vi "FeedbackDecode_UnpackPupilInfo.vi"(8 "ErrorIn":errorcluster, 11 "MSGPackStr":string="ˆ¥topic¥pupilªconfidenceË\u0000\u0000\u0000\u0000\u0000\u0000\u0000\u0000§ellipseƒ¦center’Ë\u0000\u0000\u0000\u0000\u0000\u0000\u0000\u0000Ë\u0000\u0000\u0000\u0000\u0000\u0000\u0000\u0000¤axes’Ë\u0000\u0000\u0000\u0000\u0000\u0000\u0000\u0000Ë\u0000\u0000\u0000\u0000\u0000\u0000\u0000\u0000¥angleËÀV€\u0000\u0000\u0000\u0000\u0000¨diameterË\u0000\u0000\u0000\u0000\u0000\u0000\u0000\u0000¨norm_pos’Ë\u0000\u0000\u0000\u0000\u0000\u0000\u0000\u0000Ë?ð\u0000\u0000\u0000\u0000\u0000\u0000©timestampË@µïXf¡\u001eÉ¦method¦2d c++¢id\u0000") -> (0 "ErrorOut":errorcluster, 3 "PupilClust":T1, 4 "Pupil2d":bool)   [LabVIEW 2020]
uses:
  MsgPack_LabVIEW-master/MsgPack.lvlib
panel:
  out "EmptyCnt":i32
  out "Array":variant[](array[variant])
  # "conf 8,\ndia3d 12,\nts 10\ndia 18\nmdlconf 24"
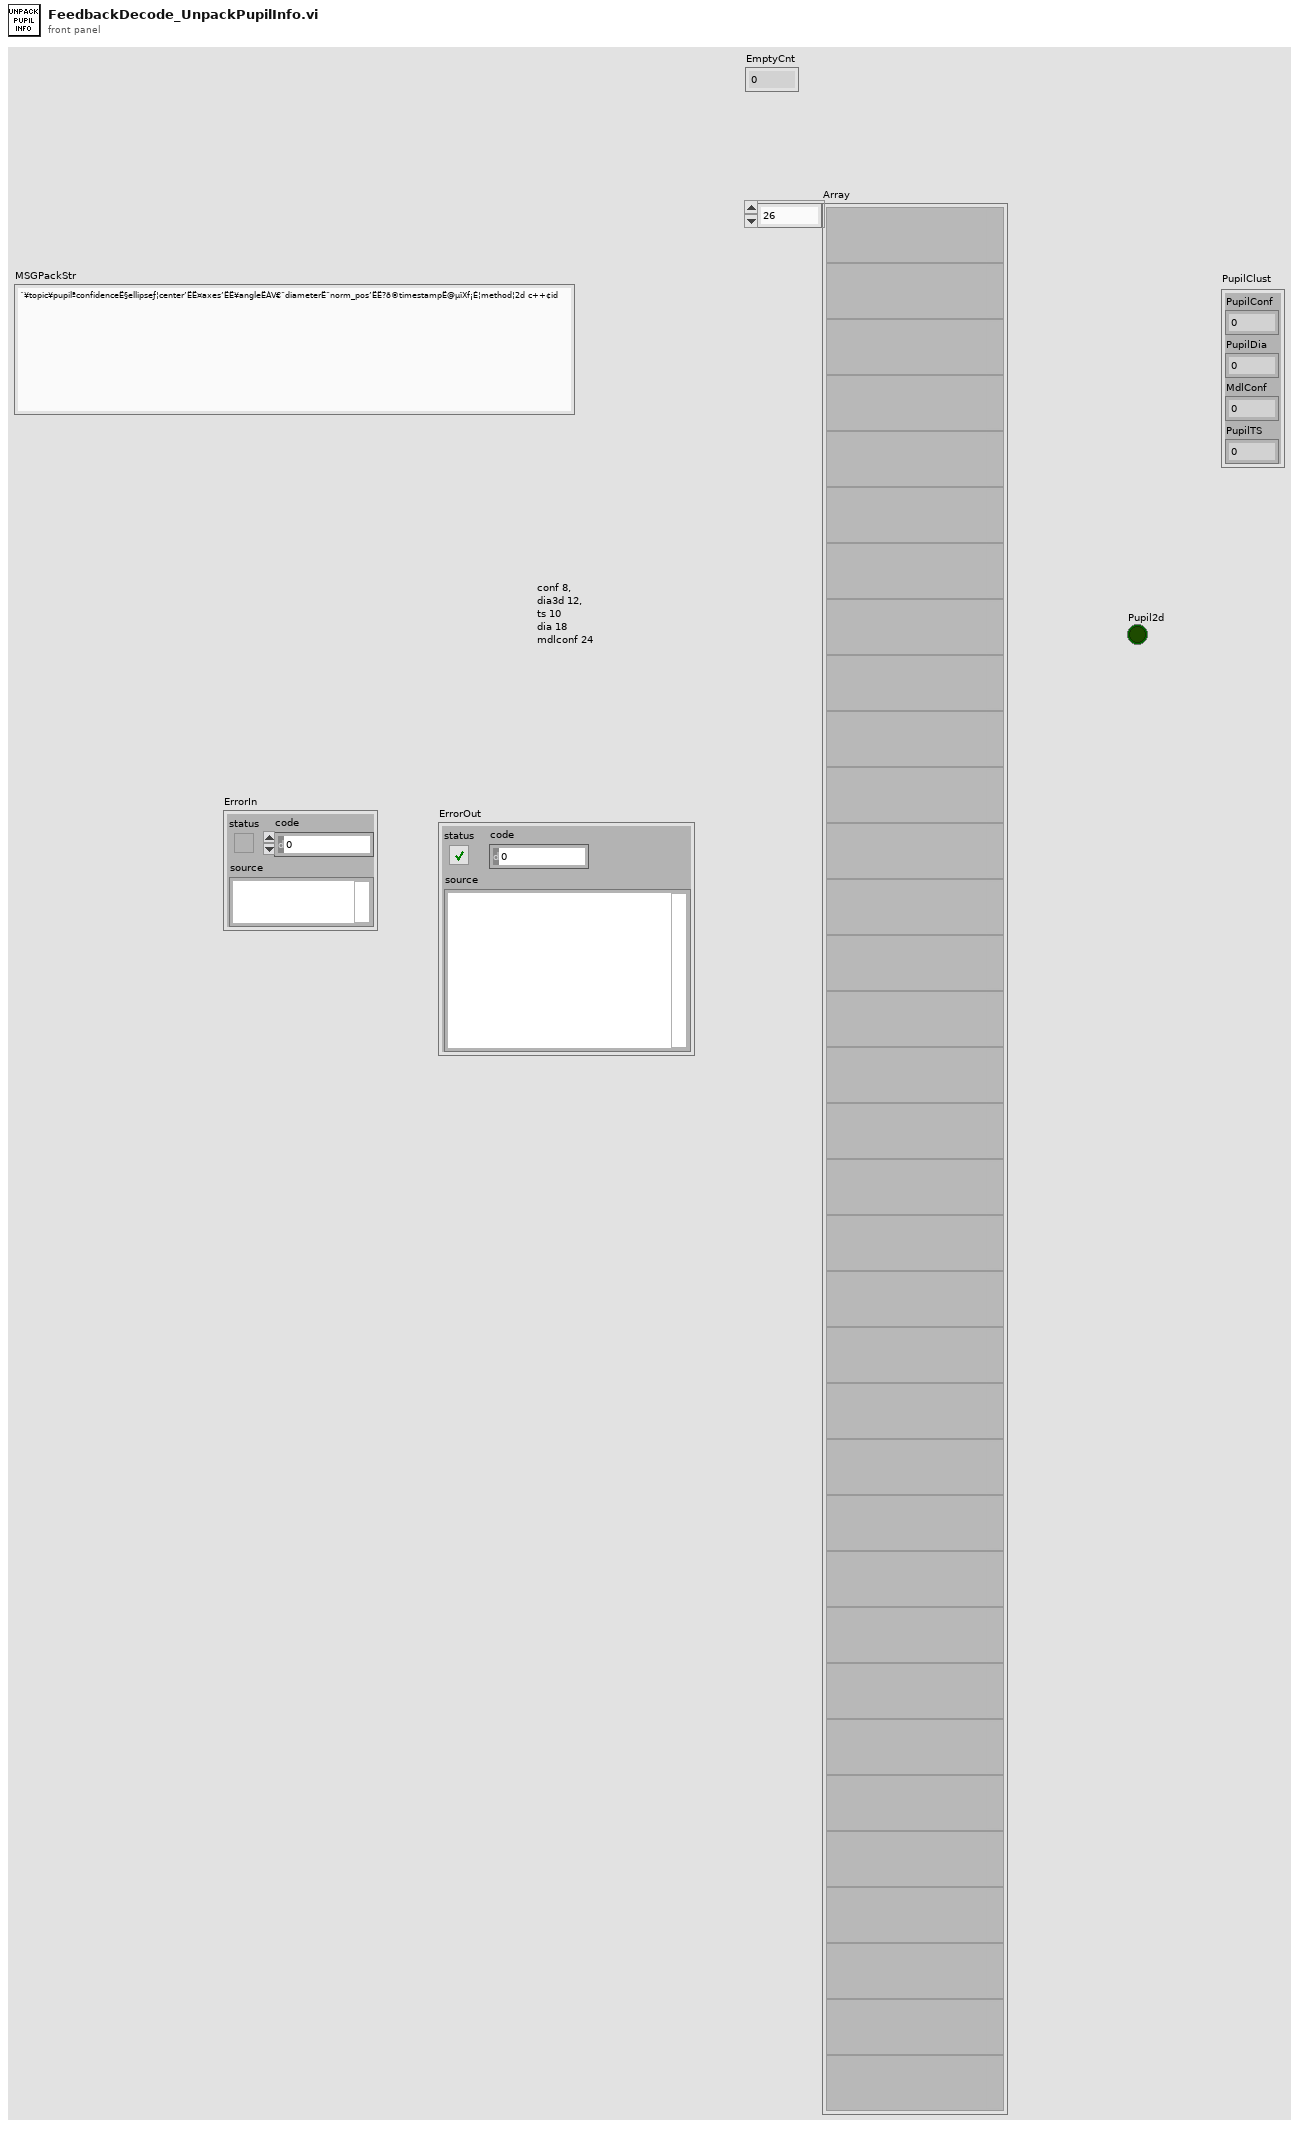
[diagram p1: front panel]
types:
  T1 = cluster{"PupilConf":dbl, "PupilDia":dbl, "MdlConf":dbl, "PupilTS":dbl}
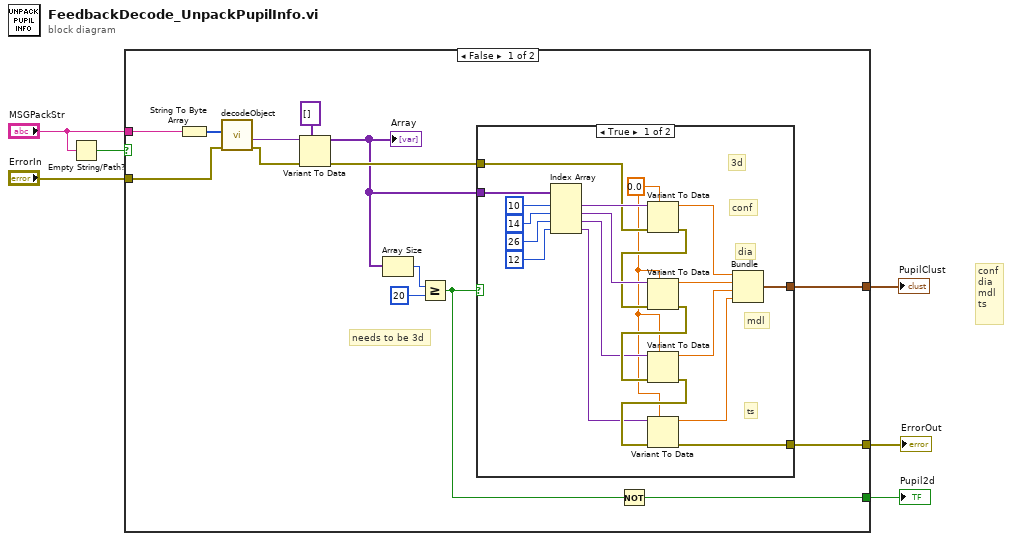
[diagram p0: block diagram]
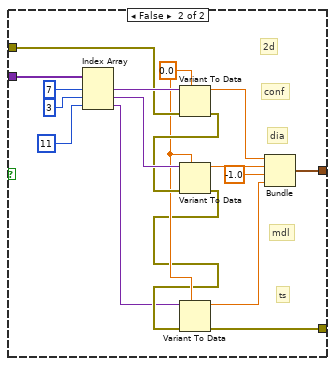
[diagram p2: hidden frame]
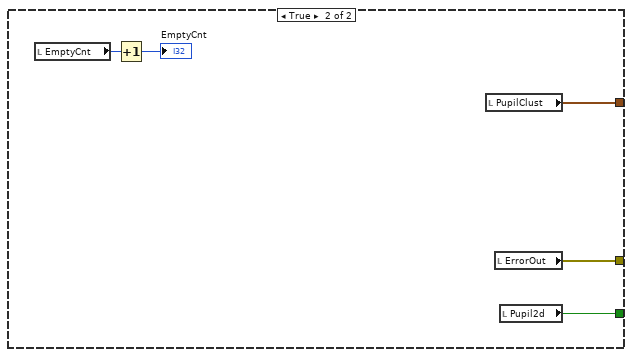
[diagram p3: hidden frame]
diagram:
  # "conf\ndia\nmdl\nts"
  n1 = Empty String/Path?(string/path="MSGPackStr") -> (empty?=w2:bool)
  n2 = case shown="False" w2 {
    tunnel: [w12 w59] -> w6
    tunnel: [w20 w60] -> w5
    tunnel: "MSGPackStr" -> [w17 _]
    tunnel: "ErrorIn" -> [w16 _]
    tunnel: [w7 w58] -> w1
    frame False {
      # "needs to be 3d"
      n3 = String To Byte Array(string=w17) -> (unsigned byte array=w13:u8[])
      n4 = call "decodeObject.vi"("error in (no error)"=w16, "ByteArray"=w13) -> ("error out"=w15:errorcluster, "Variant"=w19:variant)  [unwired: 6 in, 2 out]
      n5 = Variant To Data(error in=w15, type=variant[] [], Variant=w19) -> (data=w11:variant[], error out=w14:errorcluster)
      "Array" <- w11
      n6 = Array Size(array=w11) -> (size(s)=w10:i32)
      n7 = Greater Or Equal?(x=w10, y=20) -> (x >= y?=w8:bool)
      n8 = case shown="True" w8 {
        tunnel: [w30 w50] -> w20
        tunnel: w11 -> [w29 w49]
        tunnel: w14 -> [w28 w48]
        tunnel: [w25 w47] -> w12
        frame True {
          w24 = 0.0
          # "ts"
          # "mdl"
          # "dia"
          # "conf"
          # "3d"
          n9 = Index Array(array=w29, index #1=10 ("index"), index #2=14 ("index"), index #3=26 ("index"), index #4=12 ("index")) -> (element #1=w38:variant, element #2=w37:variant, element #3=w26:variant, element #4=w21:variant)
          n10 = Variant To Data(error in=w28, type=w24, Variant=w38) -> (data=w33:dbl, error out=w36:errorcluster)
          n11 = Variant To Data(error in=w36, type=w24, Variant=w37) -> (data=w32:dbl, error out=w34:errorcluster)
          n12 = Variant To Data(error in=w34, type=w24, Variant=w26) -> (data=w31:dbl, error out=w27:errorcluster)
          n13 = Variant To Data(error in=w27, type=w24, Variant=w21) -> (data=w23:dbl, error out=w25:errorcluster)
          n14 = Bundle(w33, w32, w31, w23) -> (w30:cluster{dbl, dbl, dbl, dbl})  [unwired: 1 in]
        }
        frame False {
          w46 = 0.0
          # "ts"
          # "mdl"
          # "dia"
          # "conf"
          # "2d"
          n15 = Index Array(array=w49, index #1=7 ("index"), index #2=3 ("index"), index #3=11 ("index")) -> (element #1=w55:variant, element #2=w54:variant, element #3=w41:variant)
          n16 = Variant To Data(error in=w48, type=w46, Variant=w55) -> (data=w52:dbl, error out=w53:errorcluster)
          n17 = Variant To Data(error in=w53, type=w46, Variant=w54) -> (data=w51:dbl, error out=w43:errorcluster)
          n18 = Variant To Data(error in=w43, type=w46, Variant=w41) -> (data=w45:dbl, error out=w47:errorcluster)
          n19 = Bundle(w52, w51, "data"=-1.0, w45) -> (w50:cluster{dbl, dbl, "data":dbl, dbl})  [unwired: 1 in]
        }
      }
      n20 = Not(x=w8) -> (.not. x?=w7:bool)
    }
    frame True {
      n21 = local read "EmptyCnt"() -> (w61:i32)
      n22 = Increment(x=w61) -> (x+1=→"EmptyCnt":i32)
      n23 = local read "PupilClust"() -> (w60:T1)
      n24 = local read "ErrorOut"() -> (w59:errorcluster)
      n25 = local read "Pupil2d"() -> (w58:bool)
    }
  }
  "ErrorOut" <- w6
  "PupilClust" <- w5
  "Pupil2d" <- w1
